vi "Remove double quotes.vi"(4 "Input string":string) -> (1 "Output string":string)   [LabVIEW 2026, in "TALOS.lvlib"]
doc: "This VI removes the double quotes in front and at the end of the string in input. Useful after getting some values (like paths) from the AEgIS Config Param."
uses:
  TALOS.lvlib
  <vilib>/Utility/error.llb/Search and Replace Pattern (string).vi
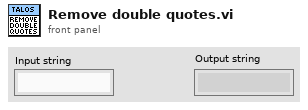
[diagram p1: front panel]
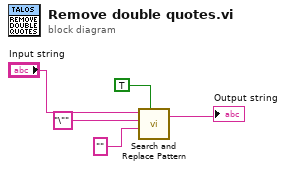
[diagram p0: block diagram]
diagram:
  n1 = call-poly <vilib>:"Search and Replace Pattern.vi"("string"="Input string", "regular expression (\"\")"="\"" ("regular expression (\"\")"), "replace string (\"\")"="" ("replace string (\"\")"), "replace all? (F)"=TRUE) -> ("result string"=→"Output string":string)  [unwired: 1 in, 1 out]
